vi "UTIL_BundleDataOut.vi"(6 "Level PV":dbl, 8 "Laser (raw)":dbl, 9 "ChB Ohms":dbl, 10 "ChA Ohms":dbl, 11 "Time (ms)":dbl) -> (0 "Level PV OUT":dbl, 1 "Measure":T1, 2 "Chart Data":T2, 3 "Data Out":dbl[](array[numeric]))   [LabVIEW 2024]
uses:
  Control Definitions/Def Measure.ctl
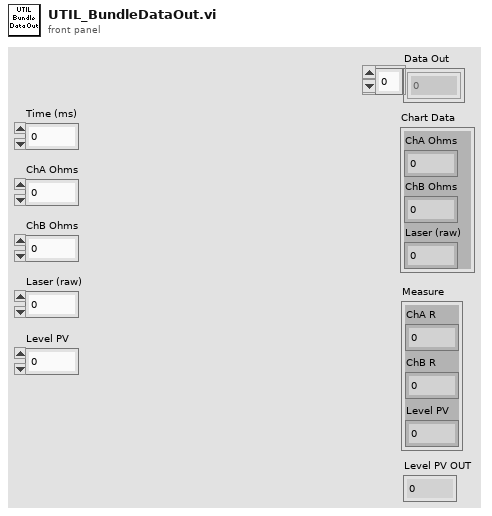
[diagram p1: front panel]
types:
  T1 = typedef "Def Measure.ctl" = cluster{"ChA R":dbl, "ChB R":dbl, "Level PV":dbl}
  T2 = cluster{"ChA Ohms":dbl, "ChB Ohms":dbl, "Laser (raw)":dbl}
  T3 = cluster{"ChA Ohms":dbl, "ChB Ohms":dbl, "Level PV":dbl}
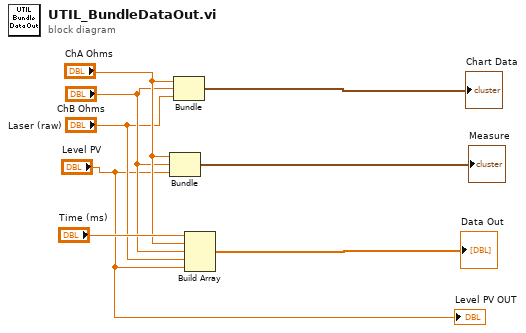
[diagram p0: block diagram]
diagram:
  n1 = Bundle("ChA Ohms"="ChA Ohms", "ChB Ohms"="ChB Ohms", "Level PV"="Level PV") -> (→"Measure":T3)  [unwired: 1 in]
  n2 = Bundle("ChA Ohms"="ChA Ohms", "ChB Ohms"="ChB Ohms", "Laser (raw)"="Laser (raw)") -> (→"Chart Data":T2)  [unwired: 1 in]
  n3 = Build Array("Time (ms)", "ChA Ohms", "ChB Ohms", "Laser (raw)", "Level PV") -> (→"Data Out":dbl[])
  "Level PV OUT" <- "Level PV"
